vi "Generate Waveforms.vi"(1 "Fade.lvclass":refnum<class "Fade.lvclass">) -> (0 "Waveforms":waveform(dbl)[](array[waveform]))   [LabVIEW 2017, in "Fade.lvclass"]
uses:
  Fade.lvclass
  C:/GitRepos/SoundDemoProject/Sound Modification/Sound Modification.lvclass
  Fade.lvclass/Fade.ctl
  Sound/Sound.lvclass
  Sound Modification/Sound Modification.lvclass
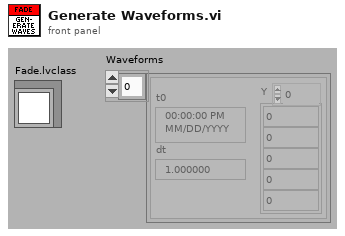
[diagram p1: front panel]
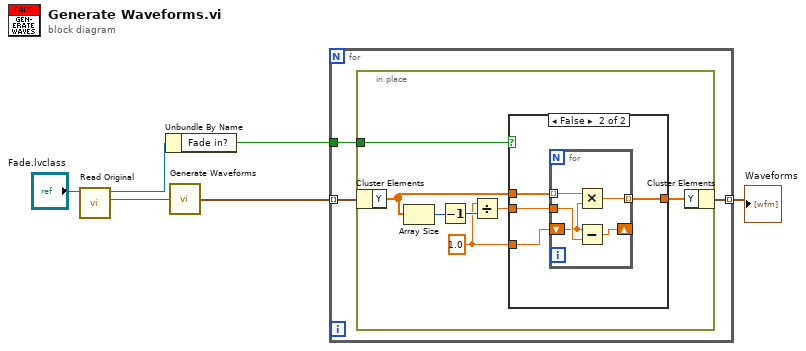
[diagram p0: block diagram]
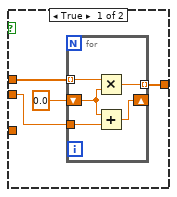
[diagram p2: hidden frame]
diagram:
  n1 = call "Read Original.vi"("Sound Modification in"="Fade.lvclass") -> ("Sound.lvclass"=w3:refnum<class "Sound.lvclass">, "Sound Modification out"=w5:refnum<class "Fade.lvclass">)  [unwired: 9 in]
  n2 = Unbundle By Name(w5) -> ("Fade in?"=w4:bool)
  n3 = call-dynamic "Generate Waveforms.vi"("Sound.lvclass"=w3) -> ("Waveforms"=w2:waveform(dbl)[])
  n4 = for {
    tunnel: w4 -> [w9]
    tunnel: w2 -> [w8] mode=indexing
    tunnel: [w7] -> w1 mode=indexing
    n5 = in-place {
      in-place-border: w9 -> [w16]
      w12 = 1.0
      n6 = in-place-cluster #1(w8) -> ("Y"=w11:dbl[])
      n7 = Array Size(array=w11) -> (size(s)=w14:i32)
      n8 = Decrement(x=w14) -> (x-1=w15:i32)
      n9 = Divide(x=w12, y=w15) -> (x/y=w13:dbl)
      n10 = case shown="False" w16 {
        tunnel: [w19 w29] -> w10
        tunnel: w13 -> [w18 w28]
        tunnel: w12 -> [_ w27]
        tunnel: w11 -> [w17 w26]
        frame True {
          n11 = for {
            shift-right: [w22] -> _
            shift-left: 0.0 -> [w23]
            tunnel: w18 -> [w24]
            tunnel: [w25] -> w19 mode=indexing
            tunnel: w17 -> [w21] mode=indexing
            n12 = Multiply(x=w21, y=w23) -> (x*y=w25:dbl)
            n13 = Add(x=w23, y=w24) -> (x+y=w22:dbl)
          }
        }
        frame False {
          n14 = for {
            shift-right: [w31] -> _
            shift-left: w27 -> [w32]
            tunnel: w28 -> [w33]
            tunnel: [w34] -> w29 mode=indexing
            tunnel: w26 -> [w30] mode=indexing
            n15 = Multiply(x=w30, y=w32) -> (x*y=w34:dbl)
            n16 = Subtract(x=w32, y=w33) -> (x-y=w31:dbl)
          }
        }
      }
      n17 = in-place-cluster #1("Y"=w10) -> (w7:waveform(dbl))
    }
  }
  "Waveforms" <- w1
